vi "Functions_String to Object.vi"(0 "scripts manager in":refnum<class "scripts manager.lvclass">, 5 "Functions":string, 7 "Line#":i64, 9 "Indent#":i64, 11 "error in (no error)":errorcluster) -> (4 "scripts manager out":refnum<class "scripts manager.lvclass">, 6 "function obj":refnum<class "functionbase.lvclass">, 8 "function created":bool, 15 "error out":errorcluster)   [LabVIEW 2016, in "scripts manager.lvclass"]
uses:
  scripts manager.lvclass
  functions/functionsbase/functionbase.lvclass
  scripts manager.lvclass/scripts manager.ctl
  functions/functionsbase/functionbase.lvclass/functionbase.ctl
  functions/functionsbase/properties/Write Func Syntax.vi
  functions/functionsbase/properties/Write Smart Syntax Representation.vi
  functions/functionsbase/properties/Write Func Full String.vi
  functions/functionsbase/properties/Write Indent#.vi
  functions/functionsbase/properties/Write Line#.vi
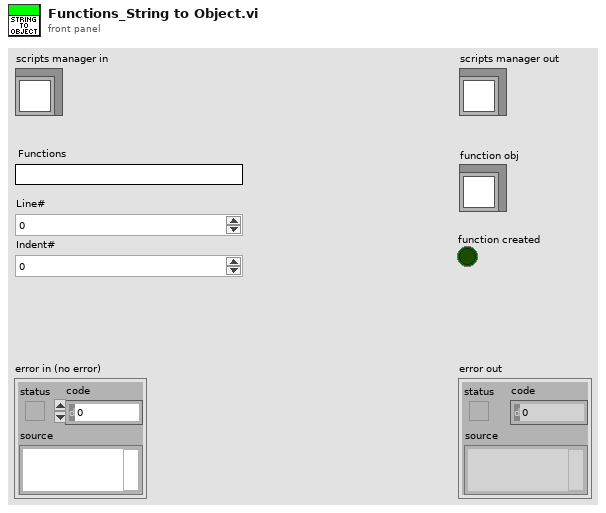
[diagram p1: front panel]
types:
  T1 = typedef "Scan Syntax Format.ctl" = cluster{"Format String":string, "Variable#":i32, "Variables Name":string[]}
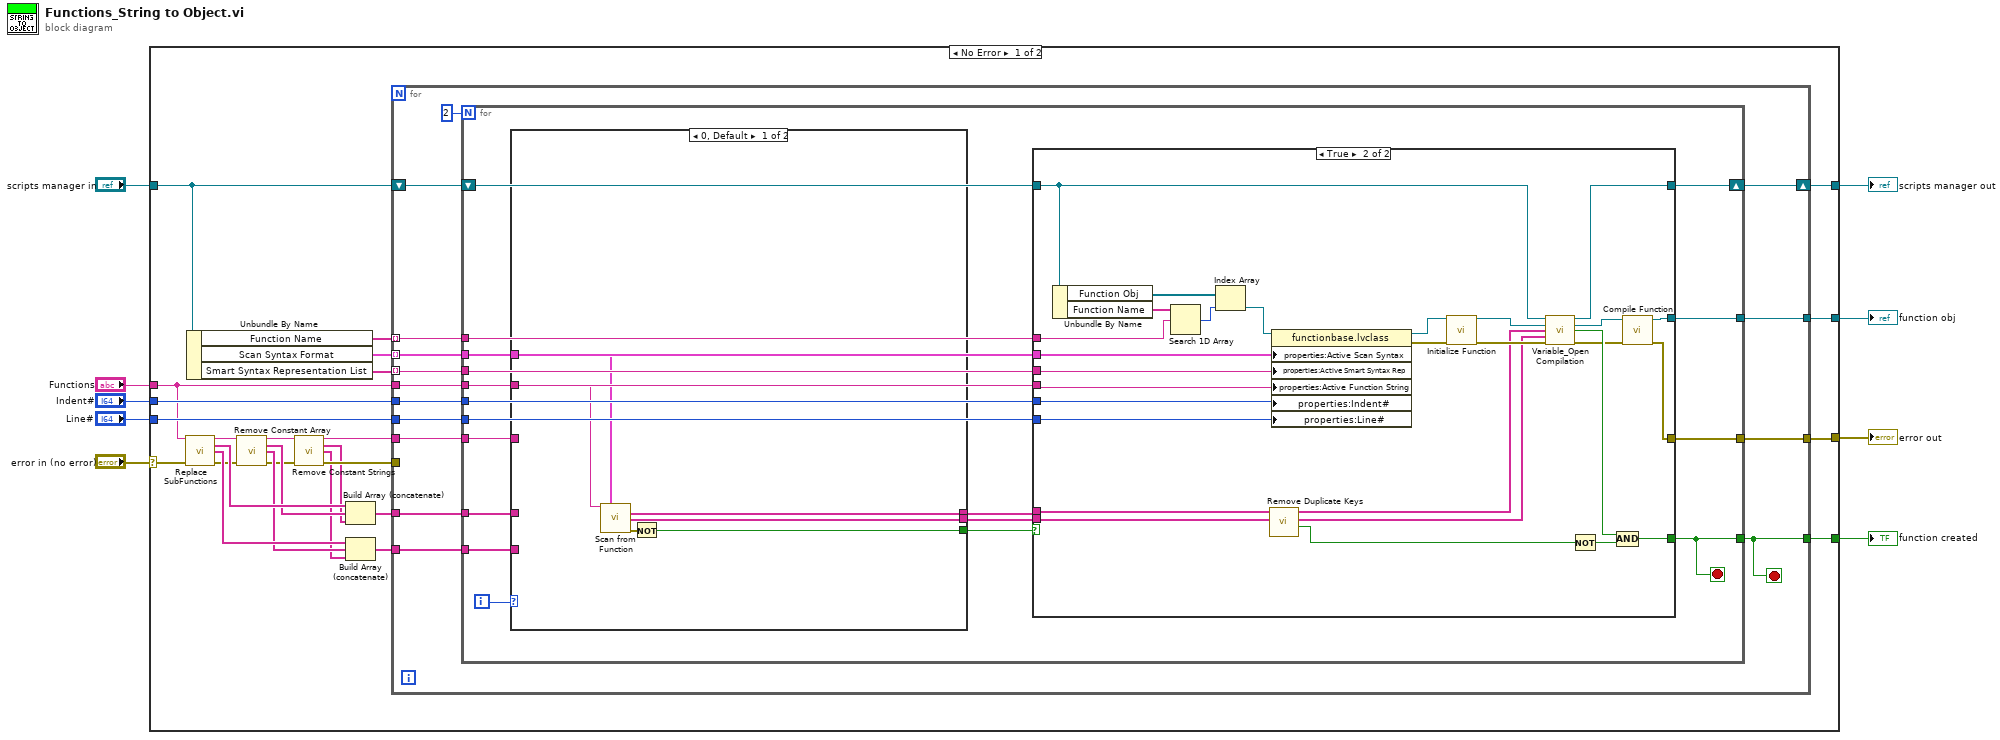
[diagram p0: block diagram]
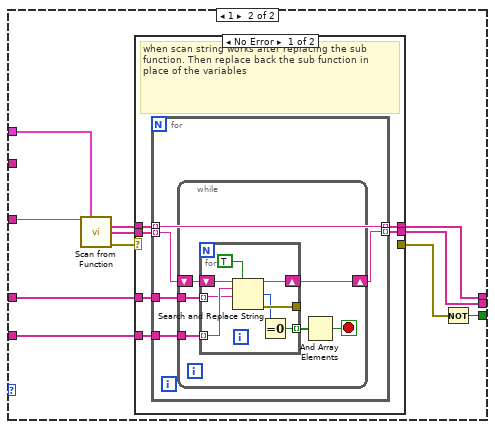
[diagram p2: hidden frame]
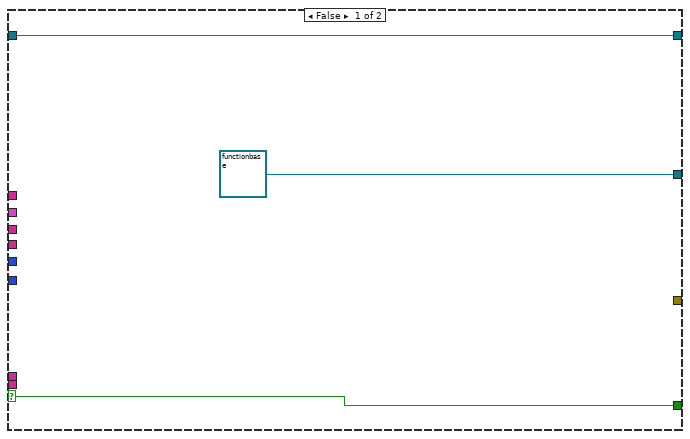
[diagram p4: hidden frame]
diagram:
  n1 = case shown="No Error" "error in (no error)" {
    selector: "error in (no error)" -> [w25 w144]
    tunnel: [w32 w144] -> w8
    tunnel: [w28 w143] -> w6
    tunnel: "scripts manager in" -> [w29 w143]
    tunnel: "Functions" -> [w22 _]
    tunnel: [w31 _] -> w4
    tunnel: [w30 _] -> w3
    tunnel: "Line#" -> [w27 _]
    tunnel: "Indent#" -> [w26 _]
    frame No Error {
      n2 = call "Replace SubFunctions.vi"("Function String"=w22, "error in (no error)"=w25) -> ("Replace Sub Function with variable"=w17:string, "Sub Functions"=w24:string[], "Variables"=w23:string[], "error out"=w16:errorcluster)  [unwired: 10 in]
      n3 = Unbundle By Name(w29) -> ("Function Name"=w34:string[], "Scan Syntax Format"=w35:T1[], "Smart Syntax Representation List"=w33:string[])
      n4 = call "Remove Constant Array.vi"("Function String"=w17, "error in (no error)"=w16) -> ("Replace Sub Function with variable"=w15:string, "Sub Functions"=w14:string[], "Variables"=w13:string[], "error out"=w12:errorcluster)  [unwired: 10 in]
      n5 = call "Remove Constant Strings.vi"("Function String"=w15, "error in (no error)"=w12) -> ("Replace Sub Function with variable"=w20:string, "Constant String"=w11:string[], "Variables"=w10:string[], "error out"=w21:errorcluster)  [unwired: 10 in]
      n6 = Build Array (concatenate)(w24, w14, w11) -> (w19:string[])
      n7 = Build Array (concatenate)(w23, w13, w10) -> (w18:string[])
      n8 = for {
        tunnel: w35 -> [w41] mode=indexing
        tunnel: w34 -> [w50] mode=indexing
        tunnel: w33 -> [w48] mode=indexing
        tunnel: w22 -> [w49]
        tunnel: w21 -> [_]
        tunnel: [w47] -> w32
        tunnel: [w46] -> w31
        tunnel: [w39] -> w30
        tunnel: w27 -> [w43]
        tunnel: w26 -> [w42]
        shift-right: [w44] -> w28
        shift-left: w29 -> [w45]
        tunnel: w20 -> [w38]
        tunnel: w19 -> [w37]
        tunnel: w18 -> [w36]
        stop <- w39 stop-if-true
        n9 = for {
          N: 2 -> [_]
          tunnel: w50 -> [w68]
          tunnel: w49 -> [w67]
          tunnel: w48 -> [w66]
          tunnel: [w65] -> w47
          tunnel: [w64] -> w46
          tunnel: w43 -> [w60]
          tunnel: w42 -> [w59]
          tunnel: w41 -> [w56]
          shift-right: [w61] -> w44
          shift-left: w45 -> [w62]
          tunnel: [w55] -> w39
          tunnel: w38 -> [w53]
          tunnel: w37 -> [w52]
          tunnel: w36 -> [w51]
          i -> [w54]
          stop <- w55 stop-if-true
          n10 = case shown="0, Default" w54 {
            tunnel: w67 -> [w74 _]
            tunnel: [w73 w78] -> w63
            tunnel: [w72 w81] -> w58
            tunnel: [w71 w80] -> w57
            tunnel: w56 -> [w69 w82]
            tunnel: w53 -> [_ w77]
            tunnel: w52 -> [_ w76]
            tunnel: w51 -> [_ w75]
            frame 0, Default {
              n11 = call "Scan from Function.vi"("initial string"=w74, "Syntax Format"=w69) -> ("Variables Name"=w72:string[], "Variables Value"=w71:string[], "error out"=w70:errorcluster)  [unwired: 10 in, 1 out]
              n12 = Not(x=w70) -> (.not. x?=w73:bool)
            }
            frame 1 {
              n13 = call "Scan from Function.vi"("initial string"=w77, "Syntax Format"=w82) -> ("Variables Name"=w84:string[], "Variables Value"=w83:string[], "error out"=w85:errorcluster)  [unwired: 10 in, 1 out]
              n14 = case shown="No Error" w85 {
                selector: w85 -> [_ w111]
                tunnel: [_ w111] -> w79
                tunnel: w84 -> [w91 _]
                tunnel: w83 -> [w90 _]
                tunnel: w76 -> [w89 _]
                tunnel: w75 -> [w88 _]
                tunnel: [w87 _] -> w81
                tunnel: [w86 _] -> w80
                frame No Error {
                  # "when scan string works after replacing the sub function. Then replace back the sub function in place of the variables"
                  n15 = for {
                    tunnel: w91 -> [w96] mode=indexing
                    tunnel: w90 -> [w93] mode=indexing
                    tunnel: w89 -> [w95]
                    tunnel: w88 -> [w94]
                    tunnel: [w96] -> w87 mode=indexing
                    tunnel: [w92] -> w86 mode=indexing
                    n16 = while {
                      tunnel: w95 -> [w102]
                      tunnel: w94 -> [w101]
                      shift-right: [w99] -> w92
                      shift-left: w93 -> [w100]
                      stop <- w97 stop-if-true
                      n17 = for {
                        tunnel: w102 -> [w106] mode=indexing
                        tunnel: w101 -> [w107] mode=indexing
                        shift-right: [w109] -> w99
                        shift-left: w100 -> [w110]
                        tunnel: [w108] -> _
                        tunnel: [w103] -> w98 mode=indexing
                        n18 = Search and Replace String(replace all?=TRUE ("replace all? (F)"), input string=w110, search string=w107, replace string=w106) -> (result string=w109:string, number of replacements=w104:i32, error out=w108:errorcluster)  [unwired: 4 in, 1 out]
                        n19 = Equal To 0?(x=w104) -> (x = 0?=w103:bool)
                      }
                      n20 = And Array Elements(Boolean array=w98) -> (logical AND=w97:bool)
                    }
                  }
                }
                frame Error {
                }
              }
              n21 = Not(x=w79) -> (.not. x?=w78:bool)
            }
          }
          n22 = case shown="True" w63 {
            selector: w63 -> [w113 _]
            tunnel: w68 -> [_ w141]
            tunnel: w56 -> [_ w137]
            tunnel: w67 -> [_ w135]
            tunnel: [_ w117] -> w65
            tunnel: [refnum<class "functionbase.lvclass"> refnum ("functionbase.lvclass") w119] -> w64
            tunnel: w66 -> [_ w136]
            tunnel: w58 -> [_ w128]
            tunnel: w57 -> [_ w127]
            tunnel: [w113 w122] -> w55
            tunnel: w62 -> [w112 w132]
            tunnel: [w112 w130] -> w61
            tunnel: w60 -> [_ w116]
            tunnel: w59 -> [_ w115]
            frame False {
            }
            frame True {
              n23 = Unbundle By Name(w132) -> ("Function Obj"=w140:refnum<class "functionbase.lvclass">[], "Function Name"=w142:string[])
              n24 = Search 1D Array(1D array=w142, element=w141) -> (index of element=w139:i32)  [unwired: 1 in]
              n25 = Index Array(array=w140, index=w139) -> (element=w138:refnum<class "functionbase.lvclass">)
              n26 = call "Remove Duplicate Keys.vi"("Variables Value in"=w127, "Variables Name in"=w128) -> ("Invalid Duplicates"=w123:bool, "Variables Value"=w125:string[], "Variables Name"=w126:string[])  [unwired: 7 in]
              n27 = property class="functionbase.lvclass"(reference=w138, "properties:Active Scan Syntax"=w137, "properties:Active Smart Syntax Rep"=w136, "properties:Active Function String"=w135, "properties:Indent#"=w115, "properties:Line#"=w116) -> (reference out=w133:refnum<class "functionbase.lvclass">, error out=w134:errorcluster)  [unwired: 1 in]
              n28 = call-dynamic "Initialize Function.vi"("functionbase in"=w133, "error in (no error)"=w134) -> ("functionbase out"=w129:refnum<class "functionbase.lvclass">, "error out"=w131:errorcluster)  [unwired: 12 in]
              n29 = call-dynamic "Variable_Open Compilation.vi"("scripts manager in"=w132, "function in"=w129, "Variables Name"=w126, "Variables Value"=w125, "error in (no error)"=w131) -> ("scripts manager out"=w130:refnum<class "scripts manager.lvclass">, "function"=w120:refnum<class "functionbase.lvclass">, "Compilation passed?"=w121:bool, "error out"=w118:errorcluster)  [unwired: 7 in]
              n30 = Not(x=w123) -> (.not. x?=w124:bool)
              n31 = Compound Arithmetic op=AND(w121, w124) -> (w122:bool)
              n32 = call-dynamic "Compile Function.vi"("error in (no error)"=w118, "functionbase in"=w120) -> ("error out"=w117:errorcluster, "functionbase out"=w119:refnum<class "functionbase.lvclass">)  [unwired: 8 in]
            }
          }
        }
      }
    }
    frame Error {
    }
  }
  "error out" <- w8
  "scripts manager out" <- w6
  "function obj" <- w4
  "function created" <- w3
